vi "transfer_zpoints_loop.vi"() -> ()   [LabVIEW 2010]
uses:
  scan_specification_cluster.ctl
panel:
  out "transferred z/intensity tuples":u32
  in  "transfer z-points?":bool
  in  "scan specification":T1={"x amplitude"=1000, "x resolution (pixels)"=200, "x offset fly-forward (iterations)"=0, "x offset fly-back (iterations)"=0, "y resolution (nr. of lines)"=200, "y step size"=5, "iterations per pixel"=5, "number of frames"=-1, "y offset (pixels)"=0, "number of y-brake lines  (before y-fly-back)"=2, "number y-brake lines (after y-fly-back)"=2, "number of y-fly-back steps"=2, "lines per z step"=0, "number of z/intensity tuples"=0}
  in  "stop":bool
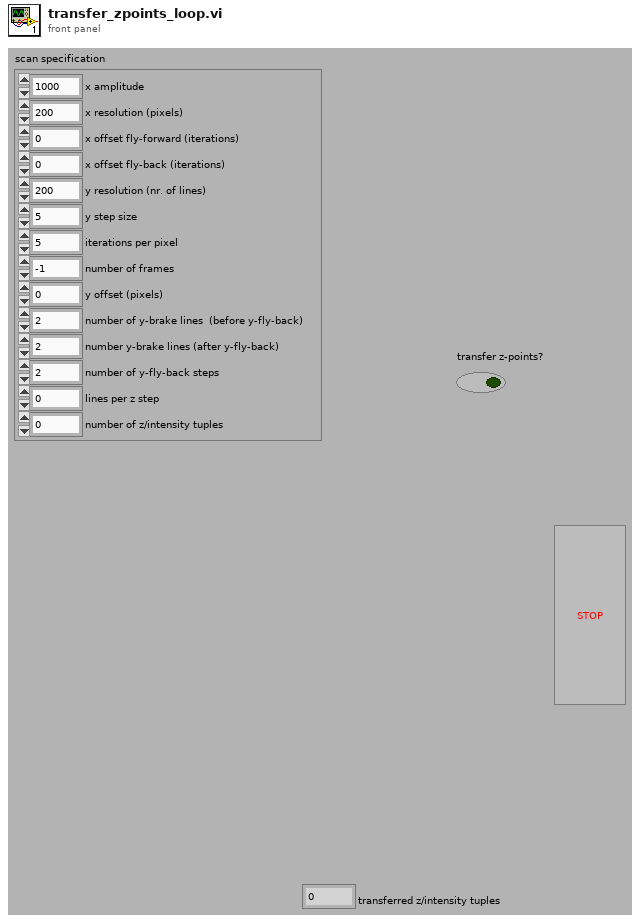
[diagram p1: front panel]
types:
  T1 = typedef "scan_specification_cluster.ctl" = cluster{"x amplitude":u16, "x resolution (pixels)":u16, "x offset fly-forward (iterations)":u16, "x offset fly-back (iterations)":u16, "y resolution (nr. of lines)":u16, "y step size":u16, "iterations per pixel":u16, "number of frames":i32, "y offset (pixels)":u16, "number of y-brake lines  (before y-fly-back)":u16, "number y-brake lines (after y-fly-back)":u16, "number of y-fly-back steps":u16, "lines per z step":u16, "number of z/intensity tuples":u16}
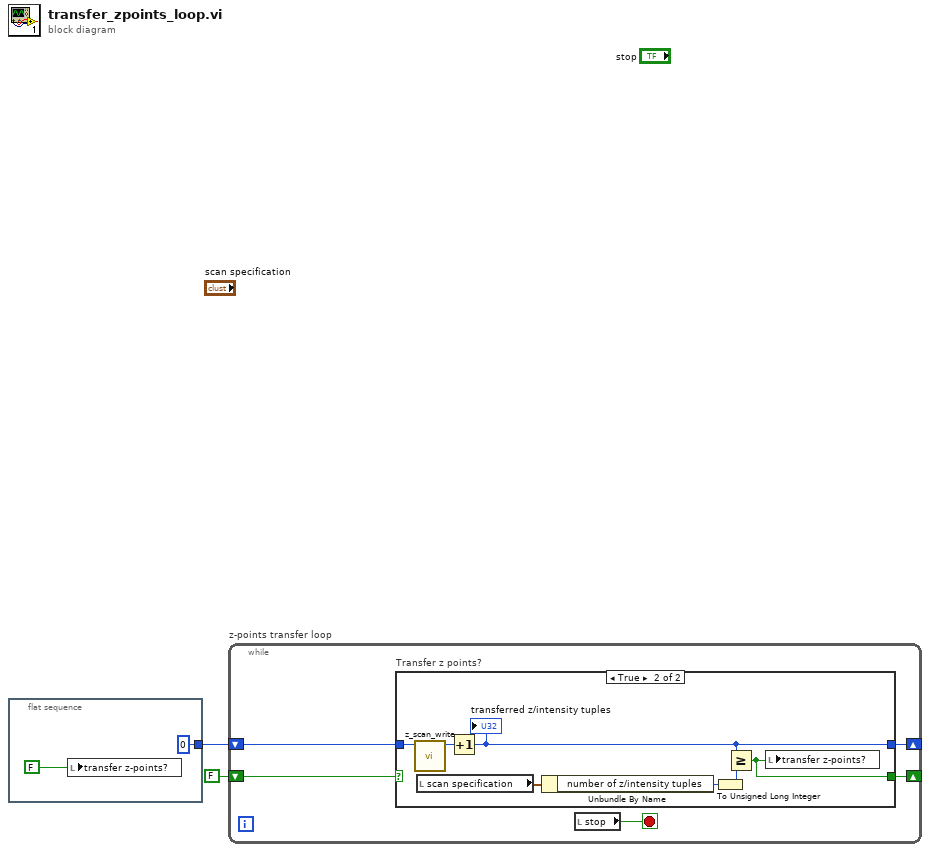
[diagram p0: block diagram]
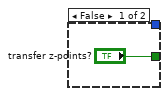
[diagram p2: hidden frame]
diagram:
  n1 = flat-sequence {
    tunnel: [u32 0 ("address out")] -> w2
    frame #0 {
      n2 = local write "transfer z-points?"(FALSE ("start z-points transfer?")) -> ()
    }
  }
  n3 = while "z-points transfer loop" {
    shift-right: [w8] -> _
    shift-left: w2 -> [w9]
    shift-right: [w6] -> _
    shift-left: FALSE ("transfer z-points?") -> [w5]
    stop <- w7 stop-if-true
    n4 = case "Transfer z points?" shown="True" w5 {
      tunnel: w9 -> [_ w17]
      tunnel: [_ w15] -> w8
      tunnel: ["transfer z-points?" w11] -> w6
      frame False {
      }
      frame True {
        n5 = call "z_scan_write.vi"("address in"=w17) -> ("address out"=w16:u32)  [unwired: 9 in, 1 out]
        n6 = local read "scan specification"() -> (w14:T1)
        n7 = Increment(x=w16) -> (x+1=w15:u32)
        "transferred z/intensity tuples" <- w15
        n8 = Unbundle By Name(w14) -> ("number of z/intensity tuples"=w13:u16)
        n9 = To Unsigned Long Integer(number=w13) -> (unsigned 32bit integer=w12:u32)
        n10 = Greater Or Equal?(x=w15, y=w12) -> (x >= y?=w11:bool)
        n11 = local write "transfer z-points?"(w11) -> ()
      }
    }
    n12 = local read "stop"() -> (w7:bool)
  }
